vi "Gobal_Progress Tracking State.vi"() -> ()   [LabVIEW 2019, in "Project.Dependencies Finder.lvlib"]
uses:
  Project.Dependencies Finder.lvlib
panel:
  out "Tracking?":bool
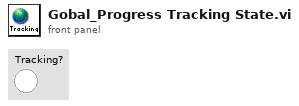
[diagram p1: front panel]
diagram:
